vi "ADAM_scan_table.vi"() -> ()   [LabVIEW 2012]
uses:
  Anemometry/Anemometry Sub Vis/Controls/Serveds.ctl
  ADAM Client/Sub VIs/ADAM Controls/Module_type_ADAM.ctl
  ADAM Client/Sub VIs/ADAM Controls/Traverse_Level_State.ctl
  Anemometry/Anemometry Sub Vis/Controls/Post_Process.ctl
  ADAM Client/Sub VIs/ADAM Controls/Channel_State.ctl
  ADAM Client/Sub VIs/ADAM Controls/Ch_description_ADAM.ctl
  ADAM Client/Sub VIs/ADAM Controls/Function_ADAM.ctl
  ADAM Client/Sub VIs/ADAM Controls/Calib_type_ADAM.ctl
  ADAM Client/Sub VIs/ADAM Controls/Address.ctl
  ADAM_Global.vi
  Sub VI's/Channel_Description_Global.vi
  Anemometry/Anemometry Sub Vis/Globals/Meas_global.vi
  Sub VI's/Logged_Data_real_Global.vi
  Anemometry/Anemometry Sub Vis/Globals/Preference_global.vi
  Anemometry/Anemometry Sub Vis/Globals/Gas_management_global.vi
  Anemometry/Anemometry Sub Vis/Globals/Constants_global.vi
panel:
  in  "Reconfigure Gills":bool
  in  "Full Res Pathname":path
  in  "Log full Res Data":bool
  out "Duty No":u16 format="%.0b"
  in  "Save Current setup":bool=TRUE
  in  "Load setup from file":bool
  out "ADAM scan comments":string
  out "History length":i32=250
  in  "stop":bool
  out "Results":dbl[](array[numeric]) format="%.3f"
  out "Titles":string[](array[string])
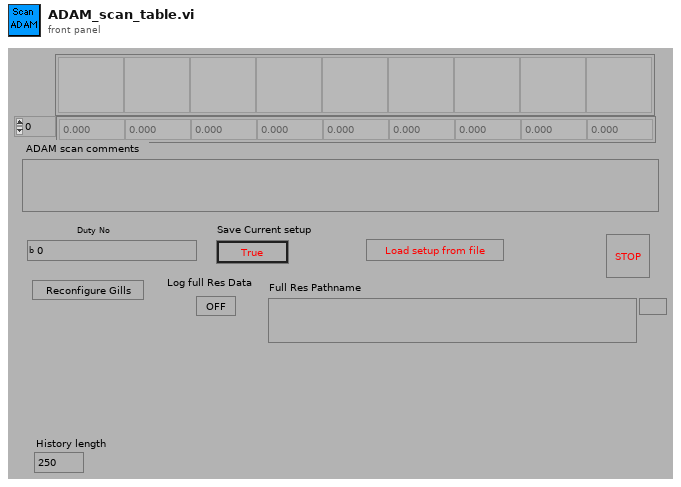
[diagram p1: front panel]
types:
  T1 = enum16{"Load ADAM setup from excel file", "Save ADAM setup to excel file"}
  T2 = typedef "Serveds.ctl" = enum16{"Read Global", "Load Global From File"}
  T3 = typedef "Module_type_ADAM.ctl" = string
  T4 = typedef "Traverse_Level_State.ctl" = enum16{"Running", "Complete"}
  T5 = typedef "Post_Process.ctl" = enum16{"Take New Data", "Post Process Raw Data File"}
  T6 = typedef "Channel_State.ctl" = enum16{"On", "Off", "Always On", "Always Off"}
  T7 = enum16{"Append to Global", "Read Global then Clear"}
  T8 = typedef "Ch_description_ADAM.ctl" = cluster{"Ch Name":string, "Type":T3, "Function":T9, "Ch State":T6, "Calibration type":T10, "A":dbl, "B":dbl, "C":dbl, "D":dbl, "Comments":string, "Address":T11, "String":string, "Duty":u16}
  T9 = typedef "Function_ADAM.ctl" = enum16{"Analogue Input", "Digital Input", "Event counter", "Event rate", "Analogue Output", "Digital Output", "Relay Output"}
  T10 = typedef "Calib_type_ADAM.ctl" = enum16{"Raw", "Bx + A", "Cx^2 + Bx + A", "Dx^3 + Cx^2 + Bx + A", "In Band", "Hi-Tec Q", "Hi-Tec M_dot", "Text"}
  T11 = typedef "Address.ctl" = cluster{"Main":i32, "Ch.":i32, "Sub":i32, "Port Name":string}
  T12 = typedef "Client_State_Cluster.ctl" = cluster{"Client Name":string, "Traverse level State":T4, "People to Email":string[], "Next Contact Time":dbl}
  T13 = typedef "ADAM_Comparitor.ctl" = cluster{"Ch to Monitor":string, "Channels to Kill":string, "Warn if Above":dbl, "Warn if Below":dbl, "Kill if Above":dbl, "Kill if Below":dbl, "Hysteresis Margin":dbl, "Averaging TIme (s)":dbl, "Warn Status":bool, "Kill Status":bool, "Extra Email addresses":string}
  T14 = typedef "Update_scan_value.ctl" = cluster{"Channel Name":string, "New Value":dbl}
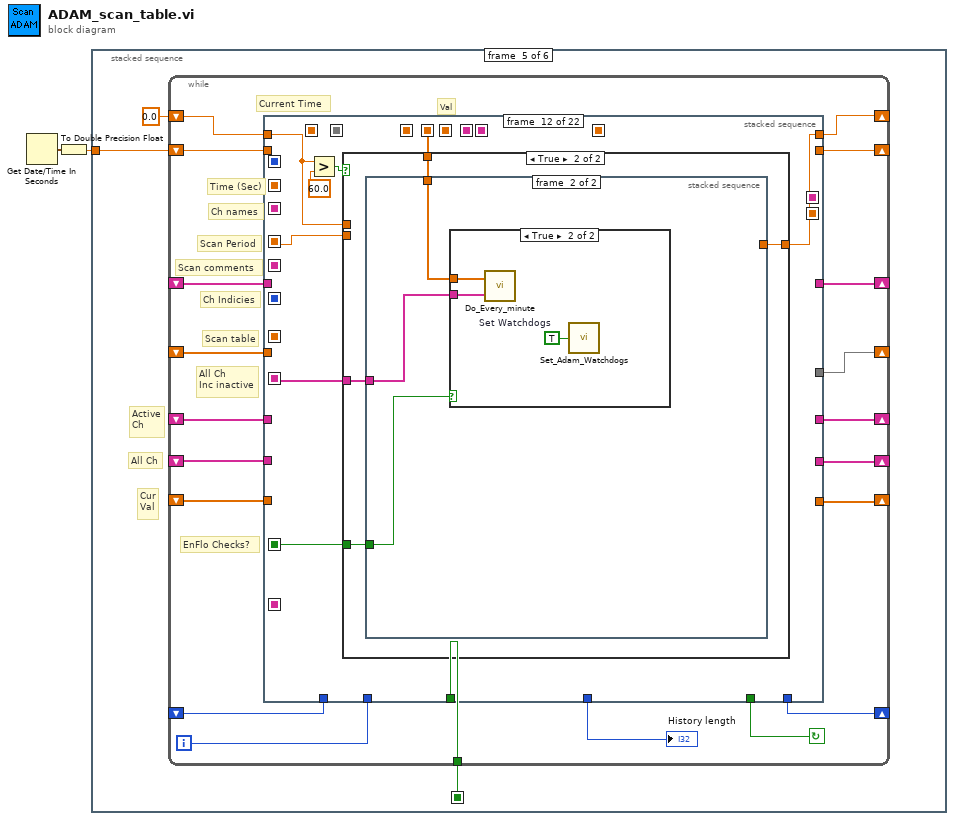
[diagram p0: block diagram]
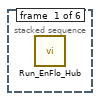
[diagram p2: hidden frame]
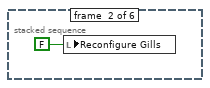
[diagram p3: hidden frame]
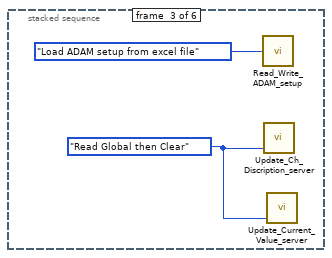
[diagram p4: hidden frame]
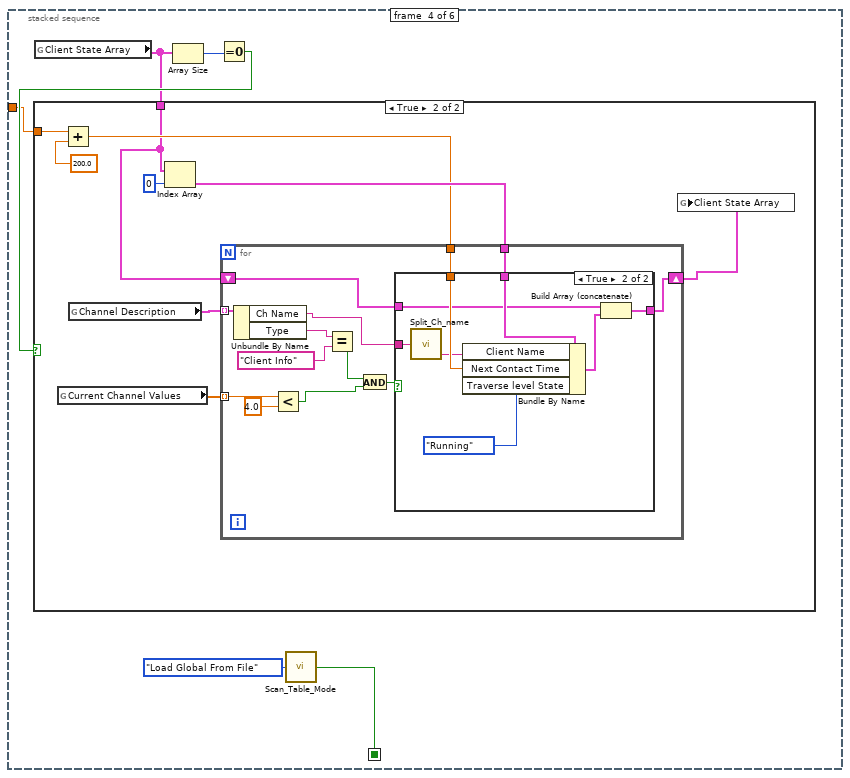
[diagram p5: hidden frame]
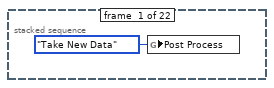
[diagram p8: hidden frame]
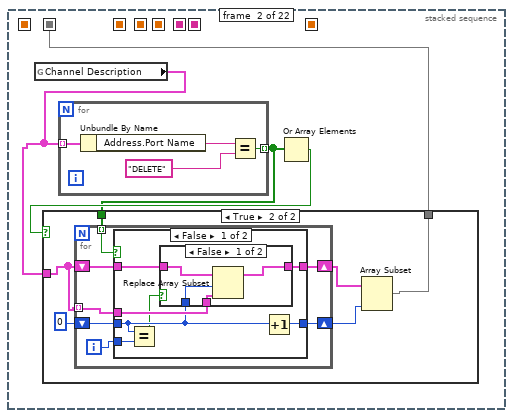
[diagram p9: hidden frame]
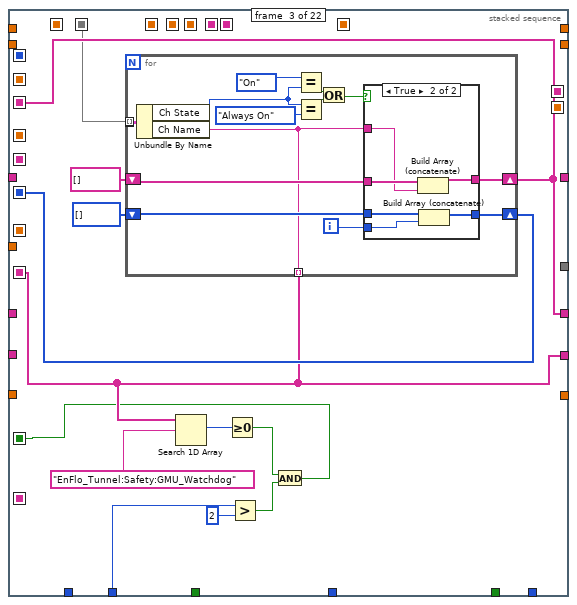
[diagram p13: hidden frame]
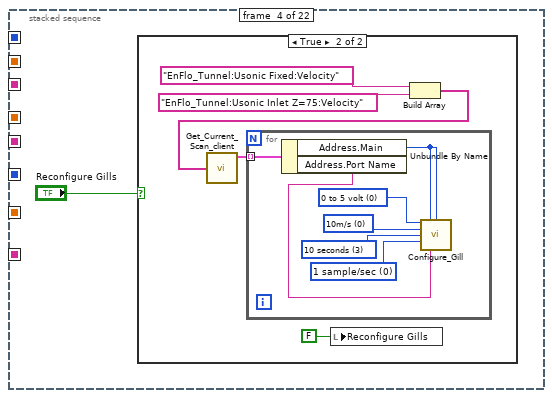
[diagram p15: hidden frame]
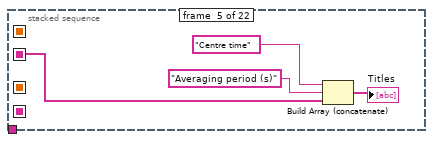
[diagram p17: hidden frame]
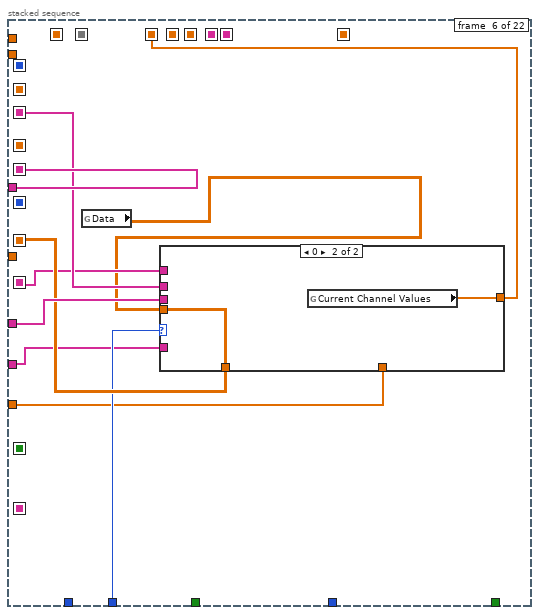
[diagram p18: hidden frame]
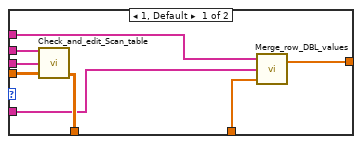
[diagram p19: hidden frame]
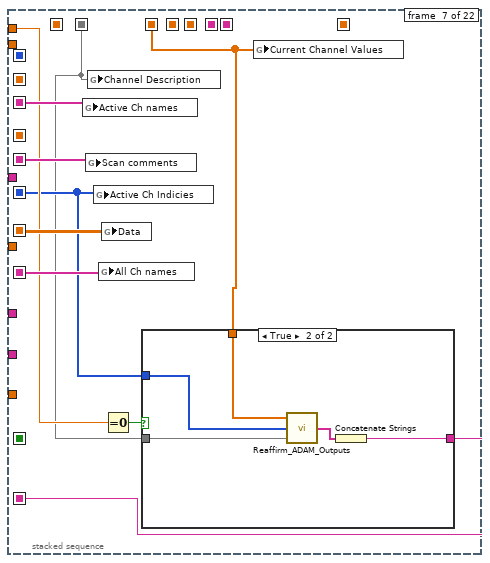
[diagram p20: hidden frame]
diagram:
  n1 = Get Date/Time In Seconds() -> (seconds since 1Jan1904=w2:timestamp)
  n2 = To Double Precision Float(number=w2) -> (double precision float=w1:dbl)
  n3 = stacked-sequence {
    seq-local: [_ _ _ w11 _ _] -> [_ _ _ _ w45 _]
    tunnel: w1 -> [_ _ _ w6 w43 _]
    frame #0 {
      n4 = call "Run_EnFlo_Hub.vi"() -> ()  [unwired: 8 out]
    }
    frame #1 {
      n5 = local write "Reconfigure Gills"(FALSE ("Reconfigure Gills")) -> ()
    }
    frame #2 {
      w4 = T7."Read Global then Clear" ("Mode")
      n6 = call "Read_Write_ADAM_setup.vi"("Mode"=T1."Load ADAM setup from excel file") -> ()  [unwired: 4 out]
      n7 = call "Update_Ch_Discription_server.vi"("Mode"=w4) -> ()  [unwired: 2 in, 1 out]
      n8 = call "Update_Current_Value_server.vi"("Mode"=w4) -> ()  [unwired: 2 in, 1 out]
    }
    frame #3 {
      n9 = global read "ADAM_Global.vi" "Client State Array"() -> (w7:T12[])
      n10 = Array Size(array=w7) -> (size(s)=w9:i32)
      n11 = Equal To 0?(x=w9) -> (x = 0?=w8:bool)
      n12 = case shown="True" w8 {
        tunnel: w7 -> [_ w13]
        tunnel: w6 -> [_ w16]
        frame False {
        }
        frame True {
          n13 = global read "ADAM_Global.vi" "Current Channel Values"() -> (w20:dbl[])
          n14 = Add(x=w16, y=200.0) -> (x+y=w14:dbl)
          n15 = global read "Channel_Description_Global.vi" "Channel Description"() -> (w19:T8[])
          n16 = Index Array(array=w13, index=0) -> (element=w17:T12)
          n17 = for {
            tunnel: w19 -> [w33] mode=indexing
            tunnel: w20 -> [w25] mode=indexing
            tunnel: w17 -> [w26]
            tunnel: w14 -> [w24]
            shift-right: [w23] -> w12
            shift-left: w13 -> [w22]
            n18 = Unbundle By Name(w33) -> ("Ch Name"=w21:string, "Type"=w30:T3)
            n19 = Less?(x=w25, y=4.0) -> (x < y?=w28:bool)
            n20 = Equal?(x=w30, y=T3 "Client Info" ("Type")) -> (x = y?=w29:bool)
            n21 = And(x=w29, y=w28) -> (x .and. y?=w27:bool)
            n22 = case shown="True" w27 {
              tunnel: w26 -> [_ w42]
              tunnel: w24 -> [_ w41]
              tunnel: [w34 w39] -> w23
              tunnel: w22 -> [w34 w38]
              tunnel: w21 -> [_ w36]
              frame False {
              }
              frame True {
                n23 = call "Split_Ch_name.vi"("Ch name"=w36) -> ("Low level"=w35:string)  [unwired: 2 out]
                n24 = Bundle By Name(cluster=w42, "Client Name"=w35, "Next Contact Time"=w41, "Traverse level State"=Traverse_Level_State."Running") -> (w37:T12)
                n25 = Build Array (concatenate)(w38, w37) -> (w39:T12[])
              }
            }
          }
          n26 = global write "ADAM_Global.vi" "Client State Array"(w12) -> ()
        }
      }
      n27 = call "Scan_Table_Mode.vi"("Mode"=Serveds."Load Global From File") -> ("Simulate Mode ?"=w11:bool)
    }
    frame #4 {
      # "Active\nCh"
      # "Cur\nVal"
      # "All Ch"
      n28 = while {
        shift-left: _ -> [w47]
        shift-right: [w46] -> _
        shift-left: _ -> [w48]
        shift-right: [w49] -> _
        shift-left: _ -> [w50]
        shift-right: [w51] -> _
        tunnel: w45 -> [w53]
        shift-left: _ -> [w56]
        shift-right: [w55] -> _
        shift-left: 0.0 -> [w57]
        shift-right: [w52] -> _
        shift-left: _ -> [w59]
        shift-right: [w60] -> _
        shift-left: _ -> [w61]
        shift-right: [w62] -> _
        shift-left: w43 -> [w63]
        shift-right: [w64] -> _
        i -> [w58]
        stop <- w65 continue-if-true
        # "Current Time"
        # "EnFlo Checks?"
        # "Val"
        # "All Ch\nInc inactive"
        # "Scan comments"
        # "Scan table"
        # "Time (Sec)"
        # "Ch Indicies"
        # "Ch names"
        # "Scan Period"
        n29 = stacked-sequence {
          seq-local: [_ _ _ _ _ _ _ _ _ _ _ _ w300 _ _ _ _ _ _ _ _ _] -> [_ _ _ _ _ _ _ _ _ _ _ _ _ _ w351 w356 _ _ _ _ w434 _]
          seq-local: [_ _ _ _ _ _ _ w193 _ _ _ _ _ _ _ _ _ _ _ _ _ _] -> [_ _ _ _ _ _ _ _ _ _ _ _ _ _ _ w363 _ _ _ _ _ _]
          seq-local: [_ _ _ _ _ w160 _ _ _ _ _ _ _ _ _ _ _ _ _ _ _ _] -> [_ _ _ _ _ _ w180 _ _ _ _ _ _ _ _ w361 _ _ _ _ _ _]
          seq-local: [_ _ _ _ _ _ _ w197 _ _ _ _ _ _ _ _ _ _ _ _ _ _] -> [_ _ _ _ _ _ _ _ _ w220 _ w266 _ _ _ w362 _ _ _ _ _ _]
          seq-local: [_ _ _ _ _ w163 _ _ _ _ _ _ _ _ _ _ _ _ _ _ _ _] -> [_ _ _ _ _ _ w182 _ _ _ _ _ _ _ _ _ _ w401 _ _ _ _]
          seq-local: [_ _ _ _ _ _ _ _ _ w218 _ _ _ _ _ _ _ _ _ _ _ _] -> [_ _ _ _ _ _ _ _ _ _ w237 _ _ _ _ _ _ _ _ _ _ _]
          seq-local: [_ _ w114 _ _ _ _ _ _ _ _ _ _ _ _ _ _ _ _ _ _ _] -> [_ _ _ _ w152 w162 w183 w198 _ _ _ _ _ _ _ w359 w364 _ _ _ _ _]
          seq-local: [_ _ w113 _ _ _ _ _ _ _ _ _ _ _ _ _ _ _ _ _ _ _] -> [_ _ _ _ _ _ w176 _ _ w219 _ _ _ _ _ _ _ _ _ _ _ _]
          seq-local: [_ _ _ _ _ w156 _ _ _ _ _ _ _ _ _ _ _ _ _ _ _ _] -> [_ _ _ _ _ _ w177 _ _ w216 _ _ _ _ _ _ _ _ _ _ _ _]
          seq-local: [_ _ _ _ _ _ _ _ _ w214 _ _ _ _ _ _ _ _ _ _ _ _] -> [_ _ _ _ _ _ _ _ _ _ w242 w265 w298 _ _ _ _ _ _ _ _ _]
          seq-local: [_ _ w109 _ _ _ _ _ _ _ _ _ _ _ _ _ _ _ _ _ _ _] -> [_ _ _ _ _ w158 w181 _ _ w215 w241 w264 w299 w324 w343 w358 _ _ _ w411 _ _]
          seq-local: [_ _ _ _ _ _ _ _ w200 _ _ _ _ _ _ _ _ _ _ _ _ _] -> [_ _ _ _ _ _ _ _ _ w213 _ _ _ _ _ _ _ _ _ _ _ _]
          seq-local: [_ w67 _ _ _ _ _ _ _ _ _ _ _ _ _ _ _ _ _ _ _ _] -> [_ _ w111 _ _ _ w175 _ _ w212 _ _ _ _ _ _ _ _ _ _ _ _]
          seq-local: [_ _ _ _ _ _ _ w192 _ _ _ _ _ _ _ _ _ _ _ _ _ _] -> [_ _ _ _ _ _ _ _ _ _ w238 _ _ _ _ _ w366 _ _ _ _ _]
          seq-local: [_ _ _ _ _ _ _ _ _ _ _ _ _ _ _ w355 _ _ _ _ _ _] -> [_ _ _ _ _ _ _ _ _ _ _ _ _ _ _ _ w365 _ _ _ _ _]
          seq-local: [_ _ w103 _ _ _ _ _ _ _ _ _ _ _ _ _ _ _ _ _ _ _] -> [_ _ _ _ _ _ _ w190 _ _ w240 w263 _ _ _ _ _ _ _ _ _ w438]
          seq-local: [_ _ _ _ _ _ _ _ _ _ _ _ w297 _ _ _ _ _ _ _ _ _] -> [_ _ _ _ _ _ _ _ _ _ _ _ _ w325 _ _ _ _ _ _ _ _]
          seq-local: [_ _ _ _ _ _ w174 _ _ _ _ _ _ _ _ _ _ _ _ _ _ _] -> [_ _ _ _ _ _ _ _ _ w211 _ _ _ _ _ _ _ _ _ _ _ _]
          seq-local: [_ _ _ _ _ _ _ _ _ _ _ _ w296 _ _ _ _ _ _ _ _ _] -> [_ _ _ _ _ _ _ _ _ _ _ _ _ w323 _ _ _ _ _ _ _ _]
          seq-local: [_ _ _ _ _ _ _ _ _ _ w236 _ _ _ _ _ _ _ _ _ _ _] -> [_ _ _ _ _ _ _ _ _ _ _ _ _ _ _ _ _ w389 _ _ _ _]
          tunnel: [_ _ _ _ _ _ _ _ _ _ _ _ _ _ _ _ _ _ w409 _ _ _] -> w65
          tunnel: [_ _ _ _ _ _ _ w192 _ _ _ _ _ _ _ _ _ _ _ _ _ _] -> w64
          tunnel: w63 -> [_ _ _ _ _ _ _ w194 _ _ _ _ _ _ _ _ _ _ _ _ _ _]
          tunnel: [_ _ _ _ _ _ _ _ _ _ _ _ _ _ _ _ _ w399 _ _ _ _] -> w62
          tunnel: w61 -> [_ _ _ _ _ w163 _ _ _ _ _ _ _ _ _ _ _ _ _ _ _ _]
          tunnel: [_ _ w114 _ _ _ _ _ _ _ _ _ _ _ _ _ _ _ _ _ _ _] -> w60
          tunnel: w59 -> [_ _ _ _ _ w161 _ _ _ _ _ _ _ w326 _ _ _ _ _ _ _ _]
          tunnel: w58 -> [_ _ w107 _ _ w159 _ _ _ _ w239 _ _ _ _ _ _ _ w407 _ _ w439]
          tunnel: w57 -> [_ _ _ _ _ _ w178 _ _ _ _ w268 _ _ _ _ _ _ _ _ _ _]
          tunnel: [_ _ _ _ _ _ _ _ _ _ _ w270 _ _ _ _ _ _ _ _ _ _] -> w52
          tunnel: w56 -> [_ _ _ _ _ _ _ _ _ _ _ _ _ _ w349 _ _ _ _ _ _ _]
          tunnel: [_ _ _ _ _ _ _ _ _ _ _ _ _ _ w345 _ _ _ _ _ _ _] -> w55
          tunnel: [_ _ _ _ _ _ _ _ _ _ _ _ _ _ _ w360 _ _ _ _ _ _] -> w54
          tunnel: w53 -> [_ _ _ _ _ _ _ _ _ w217 _ _ _ _ _ _ _ _ _ _ _ _]
          tunnel: [_ _ w109 _ _ _ _ _ _ _ _ _ _ _ _ _ _ _ _ _ _ _] -> w51
          tunnel: w50 -> [_ _ _ _ _ w157 _ _ _ _ _ _ _ _ _ _ _ _ _ _ _ _]
          tunnel: [_ _ _ _ _ _ _ _ _ _ _ _ _ _ _ _ _ _ _ _ w434 _] -> w49
          tunnel: w48 -> [_ _ _ _ _ w155 _ _ _ _ _ _ _ _ _ _ _ _ _ _ _ _]
          tunnel: w47 -> [_ _ _ _ _ _ _ _ w201 _ _ _ _ _ _ _ _ _ _ _ _ _]
          tunnel: [_ _ _ _ _ _ _ _ w202 _ _ _ _ _ _ _ _ _ _ _ _ _] -> w46
          frame #0 {
            n30 = global write "Meas_global.vi" "Post Process"(Post_Process."Take New Data" ("Post Process")) -> ()
          }
          frame #1 {
            n31 = global read "Channel_Description_Global.vi" "Channel Description"() -> (w69:T8[])
            n32 = for {
              tunnel: w69 -> [w102] mode=indexing
              tunnel: [w99] -> w68 mode=indexing
              n33 = Unbundle By Name(w102) -> ("Address.Port Name"=w101:string)
              n34 = Equal?(x=w101, y="DELETE") -> (x = y?=w99:bool)
            }
            n35 = Or Array Elements(Boolean array=w68) -> (logical OR=w70:bool)
            n36 = case shown="True" w70 {
              tunnel: w69 -> [w71 w75]
              tunnel: w68 -> [_ w77]
              tunnel: [w71 w72] -> w67
              frame False {
              }
              frame True {
                n37 = for {
                  shift-right: [w84] -> w74
                  shift-left: w75 -> [w83]
                  tunnel: w77 -> [w79] mode=indexing
                  shift-right: [w82] -> w73
                  shift-left: 0 -> [w80]
                  tunnel: w75 -> [w81] mode=indexing
                  i -> [w78]
                  n38 = case shown="False" w79 {
                    tunnel: [w90 w98] -> w84
                    tunnel: w83 -> [w91 w98]
                    tunnel: [w88 w97] -> w82
                    tunnel: w80 -> [w87 w97]
                    tunnel: w81 -> [w89 _]
                    tunnel: w78 -> [w86 _]
                    frame False {
                      n39 = Equal?(x=w87, y=w86) -> (x = y?=w85:bool)
                      n40 = case shown="False" w85 {
                        tunnel: w91 -> [w95 w96]
                        tunnel: [w94 w96] -> w90
                        tunnel: w89 -> [w93 _]
                        tunnel: w87 -> [w92 _]
                        frame False {
                          n41 = Replace Array Subset(array=w95, new element=w93, index=w92) -> (w94:T8[])
                        }
                        frame True {
                        }
                      }
                      n42 = Increment(x=w87) -> (x+1=w88:i32)
                    }
                    frame True {
                    }
                  }
                }
                n43 = Array Subset(array=w74, length=w73) -> (w72:T8[])  [unwired: 1 in]
              }
            }
          }
          frame #2 {
            n44 = for {
              tunnel: [w128] -> _ mode=indexing
              shift-right: [w127] -> w114
              shift-left: string[] [] -> [w118]
              shift-right: [w124] -> w113
              shift-left: i32[] [] -> [w126]
              tunnel: [w116] -> w109 mode=indexing
              tunnel: w111 -> [w128] mode=indexing
              i -> [w125]
              n45 = Unbundle By Name(w128) -> ("Ch State"=w119:T6, "Ch Name"=w116:string)
              n46 = Equal?(x=Channel_State."On" ("Channel State"), y=w119) -> (x = y?=w121:bool)
              n47 = Equal?(x=w119, y=Channel_State."Always On" ("Channel State")) -> (x = y?=w120:bool)
              n48 = Or(x=w121, y=w120) -> (x .or. y?=w117:bool)
              n49 = case shown="True" w117 {
                tunnel: w118 -> [w129 w136]
                tunnel: w116 -> [_ w135]
                tunnel: [w129 w134] -> w127
                tunnel: w126 -> [w130 w133]
                tunnel: w125 -> [_ w132]
                tunnel: [w130 w131] -> w124
                frame False {
                }
                frame True {
                  n50 = Build Array (concatenate)(w136, w135) -> (w134:string[])
                  n51 = Build Array (concatenate)(w133, w132) -> (w131:i32[])
                }
              }
            }
            n52 = Search 1D Array(1D array=w109, element="EnFlo_Tunnel:Safety:GMU_Watchdog") -> (index of element=w108:i32)  [unwired: 1 out]
            n53 = Greater Or Equal To 0?(x=w108) -> (x >= 0?=w104:bool)
            n54 = Greater?(x=w107, y=2) -> (0:w105:bool)
            n55 = And(x=w104, y=w105) -> (x .and. y?=w103:bool)
          }
          frame #3 {
            n56 = case shown="True" "Reconfigure Gills" {
              frame False {
              }
              frame True {
                n57 = local write "Reconfigure Gills"(FALSE ("Reconfigure Gills")) -> ()
                n58 = Build Array("EnFlo_Tunnel:Usonic Fixed:Velocity", "EnFlo_Tunnel:Usonic Inlet Z=75:Velocity") -> (w140:string[])
                n59 = call "Get_Current_Scan_client.vi"("ADAM Ch Names"=w140) -> ("Ch Description Array"=w139:T8[])  [unwired: 3 out]
                n60 = for {
                  tunnel: w139 -> [w145] mode=indexing
                  w149 = u16 0 items=["1 sample/sec", "4 samples/sec"] ("Samples/sec")
                  w148 = u16 3 items=["OFF", "3 seconds", "5 seconds", "10 seconds"] ("Averaging Time")
                  w147 = u16 0 items=["10m/s", "20m/s", "30m/s", "40m/s", "50m/s", "60m/s", "70m/s"] ("Analogue O/P Scale")
                  w146 = u16 0 items=["0 to 5 volt", "+/-2.5 Volt", "4-20mA"] ("Analogue O/P Config")
                  n61 = Unbundle By Name(w145) -> ("Address.Main"=w144:i32, "Address.Port Name"=w143:string)
                  n62 = call "Configure_Gill.vi"("Analogue O/P Config"=w146, "ORIGINAL Address"=w144, "NEW Address"=w144, "Analogue O/P Scale"=w147, "Averaging Time"=w148, "Samples/sec"=w149, "Port Name"=w143) -> ()  [unwired: 9 out]
                }
              }
            }
          }
          frame #4 {
            n63 = Build Array (concatenate)("Centre time", "Averaging period (s)", w152) -> (→"Titles":string[])
          }
          frame #5 {
            n64 = global read "Logged_Data_real_Global.vi" "Data"() -> (w154:dbl[][])
            n65 = case shown="0" w159 {
              tunnel: w154 -> [w171 w173]
              tunnel: w162 -> [w168 _]
              tunnel: w161 -> [w170 _]
              tunnel: [w169 w173] -> w160
              tunnel: w158 -> [w167 _]
              tunnel: w157 -> [w166 _]
              tunnel: [w165 w172] -> w156
              tunnel: w155 -> [w164 _]
              frame 1, Default {
                n66 = call "Check_and_edit_Scan_table.vi"("2D array input"=w171, "Original Channels"=w170, "Present Channels"=w168) -> ("2D array output"=w169:dbl[][])  [unwired: 2 out]
                n67 = call "Merge_row_DBL_values.vi"("Present Row values"=w164, "Present Channels"=w166, "Desired Channels"=w167) -> ("Desired Row values"=w165:dbl[])  [unwired: 1 out]
              }
              frame 0 {
                n68 = global read "ADAM_Global.vi" "Current Channel Values"() -> (w172:dbl[])
              }
            }
          }
          frame #6 {
            n69 = global write "ADAM_Global.vi" "Active Ch names"(w183) -> ()
            n70 = global write "ADAM_Global.vi" "Scan comments"(w182) -> ()
            n71 = global write "Channel_Description_Global.vi" "Channel Description"(w175) -> ()
            n72 = global write "ADAM_Global.vi" "Active Ch Indicies"(w176) -> ()
            n73 = global write "ADAM_Global.vi" "All Ch names"(w181) -> ()
            n74 = global write "Logged_Data_real_Global.vi" "Data"(w180) -> ()
            n75 = Equal To 0?(x=w178) -> (x = 0?=w179:bool)
            n76 = case shown="True" w179 {
              tunnel: w177 -> [_ w189]
              tunnel: w176 -> [_ w188]
              tunnel: w175 -> [_ w187]
              tunnel: ["" w185] -> w174
              frame False {
              }
              frame True {
                n77 = call "Reaffirm_ADAM_Outputs.vi"("Channel Description"=w187, "Active Ch Indicies"=w188, "Current Channel Values"=w189) -> ("Scan Comments"=w186:string[])  [unwired: 2 out]
                n78 = Concatenate Strings(w186) -> (w185:string)
              }
            }
            n79 = global write "ADAM_Global.vi" "Current Channel Values"(w177) -> ()
          }
          frame #7 {
            n80 = case shown="True" w190 {
              tunnel: w198 -> [_ w199]
              frame False {
              }
              frame True {
                n81 = call "Gas_Status_panel.vi"("Ch names"=w199) -> ()  [unwired: 15 out]
              }
            }
            n82 = Get Date/Time In Seconds() -> (seconds since 1Jan1904=w191:timestamp)
            n83 = To Double Precision Float(number=w191) -> (double precision float=w192:dbl)
            n84 = Subtract(x=w192, y=w194) -> (x-y=w197:dbl)
            n85 = Divide(x=w197, y=2.0) -> (x/y=w195:dbl)
            n86 = Add(x=w195, y=w194) -> (x+y=w193:dbl)
          }
          frame #8 {
            n87 = Equal To 0?(x=w201) -> (x = 0?=w205:bool)
            n88 = Equal?(x=u16 32768, y=w201) -> (x = y?=w204:bool)
            n89 = Select(t=u16 1, s=w205, f=w201) -> (s? t:f=w200:u16)
            "Duty No" <- w200
            n90 = case shown="False" w204 {
              tunnel: [w207 u16 0] -> w202
              tunnel: w200 -> [w209 _]
              frame False {
                n91 = Multiply(x=u16 2, y=w209) -> (x*y=w207:u16)
              }
              frame True {
              }
            }
          }
          frame #9 {
            n92 = for {
              tunnel: w212 -> [w227]
              tunnel: w220 -> [w235]
              shift-right: [w233] -> w214
              shift-left: w216 -> [w231]
              tunnel: w215 -> [w232]
              shift-right: [w228] -> w218
              shift-left: w211 -> [w230]
              tunnel: w219 -> [w222] mode=indexing
              tunnel: w216 -> [w224]
              tunnel: w217 -> [w225]
              tunnel: w213 -> [w221]
              n93 = Index Array(array=w224, index=w222) -> (element=w223:dbl)
              n94 = Index Array(array=w227, index=w222) -> (element=w226:T8)
              n95 = call "Adam_Ch_Input_Output.vi"("Simulate"=w225, "Duty No"=w221, "Previuos Scan Value"=w223, "Ch values"=w231, "Scan Period"=w235, "Ch Discription"=w226, "Ch names"=w232) -> ("Scan comment"=w229:string, "Calibrated units"=w234:dbl)  [unwired: 1 in, 2 out]
              n96 = Concatenate Strings(w230, w229) -> (w228:string)
              n97 = Replace Array Subset(array=w231, new element=w234, index=w222) -> (w233:dbl[])
            }
          }
          frame #10 {
            n98 = case shown="True" w240 {
              tunnel: w242 -> [_ w249]
              tunnel: w241 -> [_ w248]
              tunnel: w239 -> [_ w247]
              tunnel: w238 -> [_ w257]
              tunnel: w237 -> [w244 w246]
              tunnel: [w244 w254] -> w236
              frame False {
              }
              frame True {
                n99 = global read "ADAM_Global.vi" "Comparitor Array"() -> (w253:T13[])
                n100 = for {
                  tunnel: w253 -> [w262] mode=indexing
                  tunnel: [w261] -> w252 mode=indexing
                  tunnel: w249 -> [w260]
                  tunnel: w248 -> [w259]
                  tunnel: [w258] -> w251 mode=indexing
                  n101 = call "ADAM_Comparitor.vi"("Comparator Info"=w262, "Ch names"=w259, "Present scan array"=w260) -> ("Comparator Info Out"=w261:T13, "Scan comment"=w258:string)  [unwired: 1 in]
                }
                n102 = call "LDA1_Safety.vi"("Adam Loop Count"=w247, "Ch Names"=w248, "Values"=w249) -> ("Scan comment"=w245:string)
                n103 = call "LDA2_Safety.vi"("Adam Loop Count"=w247, "Ch Names"=w248, "Values"=w249) -> ("Scan comment"=w250:string)
                n104 = call "Safety_Check.vi"("Adam Loop Count"=w247, "Ch Names"=w248, "Values"=w249) -> ("Scan comment"=w256:string)
                n105 = call "Check_Aero_Tunnel_on_Server.vi"("Values"=w249, "Ch Names"=w248, "Current Time"=w257, "Adam Loop Count"=w247) -> ("Scan comment"=w255:string)  [unwired: 2 in]
                n106 = global write "ADAM_Global.vi" "Comparitor Array"(w252) -> ()
                n107 = Concatenate Strings(w246, w245, w250, w256, w255, w251) -> (w254:string)
              }
            }
            n108 = property on="Results" class="Arr (strict)"() -> ("Index Values"=w243:u32[])  [unwired: 2 in, 2 out]
            n109 = property on="Titles" class="Arr (strict)"("Index Values"=w243) -> ()  [unwired: 2 in, 2 out]
          }
          frame #11 {
            n110 = Greater?(x=w268, y=60.0) -> (0:w269:bool)
            n111 = case shown="True" w269 {
              tunnel: [w272 w277] -> w270
              tunnel: w268 -> [w273 _]
              tunnel: w266 -> [w271 _]
              tunnel: w265 -> [_ w276]
              tunnel: w264 -> [_ w275]
              tunnel: w263 -> [_ w274]
              frame False {
                n112 = Add(x=w273, y=w271) -> (x+y=w272:dbl)
              }
              frame True {
                n113 = stacked-sequence {
                  tunnel: [0.0 _] -> w277
                  tunnel: w276 -> [_ w292]
                  tunnel: w275 -> [_ w291]
                  tunnel: w274 -> [_ w290]
                  frame #0 {
                    n114 = case shown="False" "Save Current setup" {
                      tunnel: [FALSE w282] -> w278
                      frame False {
                      }
                      frame True {
                        n115 = Get Date/Time In Seconds() -> (seconds since 1Jan1904=w284:timestamp)
                        n116 = global read "ADAM_Global.vi" "Network Last checked"() -> (w288:dbl)
                        n117 = To Double Precision Float(number=w284) -> (double precision float=w283:dbl)
                        n118 = Subtract(x=w288, y=w283) -> (x-y=w287:dbl)
                        n119 = Absolute Value(x=w287) -> (abs(x)=w286:dbl)
                        n120 = Less?(x=w286, y=1.5) -> (x < y?=w282:bool)
                      }
                    }
                    n121 = case shown="True" w278 {
                      frame False {
                      }
                      frame True {
                        n122 = call "Read_Write_ADAM_setup.vi"("Mode"=T1."Save ADAM setup to excel file") -> ()  [unwired: 4 out]
                      }
                    }
                  }
                  frame #1 {
                    n123 = case shown="True" w290 {
                      tunnel: w292 -> [_ w295]
                      tunnel: w291 -> [_ w294]
                      frame False {
                      }
                      frame True {
                        w293 = TRUE  # Set Watchdogs
                        n124 = call "Do_Every_minute.vi"("Ch Names"=w294, "Values"=w295) -> ()  [unwired: 1 out]
                        n125 = call "Set_Adam_Watchdogs.vi"("Set Watchdogs"=w293) -> ()  [unwired: 1 out]
                      }
                    }
                  }
                }
              }
            }
          }
          frame #12 {
            n126 = call "Update_Current_Value_server.vi"("Mode"=T7."Read Global then Clear") -> ("Update array out"=w302:T14[])  [unwired: 2 in]
            n127 = for {
              tunnel: w299 -> [w310]
              tunnel: w302 -> [w305] mode=indexing
              shift-right: [w308] -> w300
              shift-left: w298 -> [w309]
              tunnel: [w304] -> w297 mode=indexing
              tunnel: [w303] -> w296 mode=indexing
              n128 = Unbundle By Name(w305) -> ("Channel Name"=w304:string, "New Value"=w303:dbl)
              n129 = Search 1D Array(1D array=w310, element=w304) -> (index of element=w307:i32)  [unwired: 1 out]
              n130 = Less Than 0?(x=w307) -> (x < 0?=w306:bool)
              n131 = case shown="True" w306 {
                tunnel: w304 -> [_ w311]
                tunnel: w305 -> [_ w316]
                frame False {
                }
                frame True {
                  n132 = global read "ADAM_Global.vi" "Update Current Value"() -> (w315:T14[])
                  n133 = call "Check_Ch_Name_colons.vi"("No of Colons"=2, "Ch Name in"=w311) -> ("Ch Name out"=w312:string)
                  n134 = Bundle By Name(cluster=T8 {"Ch Name"="", "Type"="Hold Value", "Function"=enum."Analogue Input", "Ch State"=enum."On", "Calibration type"=enum."Raw", "A"=0.0, "B"=0.0, "C"=0.0, "D"=0.0, "Comments"="", "Address"={"Main"=0, "Ch."=0, "Sub"=0, "Port Name"=""}, "String"="", "Duty"=0} ("Ch Description"), "Ch Name"=w312, "Type"=T3 "Hold Value") -> (w320:T8)
                  n135 = Build Array (concatenate)(w315, w316) -> (w314:T14[])
                  n136 = global write "ADAM_Global.vi" "Update Current Value"(w314) -> ()
                  n137 = global read "Preference_global.vi" "Rig Setup"() -> (w318:string)
                  n138 = Build Array(w320) -> (w319:T8[])
                  n139 = call "Update_Ch_Discription_server.vi"("Mode"=T7."Append to Global", "Client HD name"=w318, "Channels to update In"=w319) -> ()  [unwired: 1 out]
                }
              }
              n140 = Replace Array Subset(array=w309, new element=w303, index=w307) -> (w308:dbl[])
            }
          }
          frame #13 {
            n141 = for {
              tunnel: w326 -> [w334]
              tunnel: w325 -> [w332] mode=indexing
              tunnel: w324 -> [w333]
              tunnel: w323 -> [w330] mode=indexing
              n142 = Search 1D Array(1D array=w334, element=w332) -> (index of element=w331:i32)  [unwired: 1 out]
              n143 = Less Than 0?(x=w331) -> (x < 0?=w329:bool)
              n144 = Not Equal To 0?(x=w330) -> (x != 0?=w328:bool)
              n145 = And(x=w328, y=w329) -> (x .and. y?=w327:bool)
              n146 = case shown="True" w327 {
                tunnel: w333 -> [_ w342]
                tunnel: w332 -> [_ w341]
                frame False {
                }
                frame True {
                  n147 = Search 1D Array(1D array=w342, element=w341) -> (index of element=w336:i32)  [unwired: 1 out]
                  n148 = global read "Channel_Description_Global.vi" "Channel Description"() -> (w337:T8[])
                  n149 = Index Array(array=w337, index=w336) -> (element=w340:T8)
                  n150 = Bundle By Name(cluster=w340, "Ch State"=Channel_State."On") -> (w338:T8)
                  n151 = Replace Array Subset(array=w337, new element=w338, index=w336) -> (w335:T8[])
                  n152 = global write "Channel_Description_Global.vi" "Channel Description"(w335) -> ()
                }
              }
            }
          }
          frame #14 {
            n153 = Search 1D Array(1D array=w343, element="GMU:Source:Release Temp") -> (index of element=w350:i32)  [unwired: 1 out]
            n154 = Index Array(array=w351, index=w350) -> (element=w348:dbl)
            n155 = Build Array (concatenate)(w348, w349) -> (w347:dbl[])
            n156 = Array Subset(array=w347, length=10 ("Array Length")) -> (w345:dbl[])  [unwired: 1 in]
            n157 = call "Mean_fr_NaN_data.vi"("Data"=w345) -> ("Mean value"=w344:dbl)  [unwired: 1 out]
            n158 = global write "Gas_management_global.vi" "Release temp (deg C)"(w344) -> ()
          }
          frame #15 {
            w353 = 250000  # Table size
            n159 = call "Merge_row_DBL_values.vi"("Present Row values"=w356, "Present Channels"=w358, "Desired Channels"=w359) -> ("Desired Row values"=w357:dbl[])  [unwired: 1 out]
            n160 = Build Array (concatenate)(w363, w362, w357) -> (w355:dbl[])
            "Results" <- w355
            n161 = call "Manipulate_Table.vi"("Table size"=w353, "Latest Row"=w355, "Table Input"=w361) -> ("History length"=w360:i32, "Table Output"=w354:dbl[][])  [unwired: 1 out]
            n162 = global write "Logged_Data_real_Global.vi" "Data"(w354) -> ()
          }
          frame #16 {
            n163 = case shown="True" "Log full Res Data" {
              tunnel: w366 -> [_ w379]
              tunnel: w365 -> [_ w378]
              tunnel: w364 -> [_ w377]
              frame False {
              }
              frame True {
                n164 = Build Array (concatenate)(w379, w378) -> (w376:dbl[])
                n165 = Number To Fractional String(number=w376) -> (F-format string=w374:string[])  [unwired: 3 out]
                n166 = call "Does_file_exist_(simple).vi"("Pathname"="Full Res Pathname") -> ("exists?"=w373:bool)
                n167 = Build Array (concatenate)("Current time", "Centre Time", "Averaging period (s)", w377) -> (w375:string[])
                n168 = case shown="False" w373 {
                  tunnel: w375 -> [w385 _]
                  tunnel: w374 -> [w384 w386]
                  tunnel: [w381 w387] -> w369
                  frame False {
                    n169 = Build Array(w385, w384) -> (w382:string[][])
                    n170 = Array To Spreadsheet String(array=w382, 3:"%s" ("format string")) -> (spreadsheet string=w381:string)  [unwired: 1 out]
                  }
                  frame True {
                    n171 = Array To Spreadsheet String(array=w386, 3:"%s" ("format string")) -> (spreadsheet string=w387:string)  [unwired: 1 out]
                  }
                }
                n172 = call "Write_File_Simple.vi"("append to file? (new file:F)"=TRUE, "character string"=w369, "file path"="Full Res Pathname") -> ()  [unwired: 2 out]
              }
            }
          }
          frame #17 {
            w397 = 150 ("length")
            w398 = 50  # History length
            n173 = String Subset(string=w389, length (rest)=w397) -> (substring=w391:string)  [unwired: 1 out]
            n174 = String Length(string=w391) -> (length=w396:i32)
            n175 = Equal?(x=w397, y=w396) -> (x = y?=w395:bool)
            n176 = Select(t=" Clipped ", s=w395, f="") -> (s? t:f=w392:string)
            n177 = Concatenate Strings(w392, w391) -> (w390:string)
            n178 = Build Array (concatenate)(w401, w390) -> (w400:string[])
            n179 = Array Size(array=w400) -> (size(s)=w403:i32)
            n180 = Subtract(x=w403, y=w398) -> (x-y=w402:i32)
            n181 = Array Subset(array=w400, index=w402) -> (w399:string[])  [unwired: 1 in]
            "ADAM scan comments" <- w389
          }
          frame #18 {
            n182 = Format Into String(format string="%s %d %s" ("Format String"), "\nScan No " ("Header message"), w407, "\r\n") -> (resulting string=w406:string)  [unwired: 2 in, 1 out]
            n183 = call "Write_out_serial_log.vi"("Header message"=w406) -> ()
            n184 = Not(x="stop") -> (.not. x?=w409:bool)
          }
          frame #19 {
            n185 = call "Update_Ch_Discription_server.vi"("Mode"=T7."Read Global then Clear") -> ("Channels to update Out"=w412:T8[])  [unwired: 2 in]
            n186 = Array Size(array=w412) -> (size(s)=w414:i32)
            n187 = Equal To 0?(x=w414) -> (x = 0?=w413:bool)
            n188 = case shown="False" w413 {
              tunnel: w411 -> [w419 _]
              tunnel: w412 -> [w418 _]
              frame False {
                n189 = global read "Channel_Description_Global.vi" "Channel Description"() -> (w417:T8[])
                n190 = for {
                  tunnel: w419 -> [w426]
                  tunnel: w418 -> [w423] mode=indexing
                  shift-right: [w422] -> w416
                  shift-left: w417 -> [w425]
                  n191 = Unbundle By Name(w423) -> ("Ch Name"=w424:string)
                  n192 = Search 1D Array(1D array=w426, element=w424) -> (index of element=w420:i32)  [unwired: 1 out]
                  n193 = Less Than 0?(x=w420) -> (x < 0?=w421:bool)
                  n194 = case shown="False" w421 {
                    tunnel: w425 -> [w430 w433]
                    tunnel: w423 -> [w429 w431]
                    tunnel: [w428 w432] -> w422
                    tunnel: w420 -> [w427 _]
                    frame False {
                      n195 = Replace Array Subset(array=w430, new element=w429, index=w427) -> (w428:T8[])
                    }
                    frame True {
                      n196 = Build Array (concatenate)(w433, w431) -> (w432:T8[])
                    }
                  }
                }
                n197 = global write "Channel_Description_Global.vi" "Channel Description"(w416) -> ()
              }
              frame True {
              }
            }
          }
          frame #20 {
            n198 = case shown="True" "Load setup from file" {
              frame False {
              }
              frame True {
                n199 = local write "Save Current setup"(TRUE ("Save Current setup")) -> ()
                n200 = call "Read_Write_ADAM_setup.vi"("Mode"=T1."Load ADAM setup from excel file") -> ()  [unwired: 4 out]
              }
            }
          }
          frame #21 {
            n201 = case shown="0" w439 {
              tunnel: w438 -> [_ _]
              frame 0 {
                n202 = global read "Constants_global.vi" "EnFlo SW Folder"() -> (w444:path)
                n203 = Build Path(base path=w444, name or relative path=path "ADAM Client/ADAM client VIs/Plot_Server_Data.vi") -> (appended path=w441:path)
                n204 = call "Load_Comparitor_Cluster.vi"() -> ()  [unwired: 12 in]
                n205 = Build Path(base path=w444, name or relative path=path "ADAM Server/Log_ADAM_scan_table.vi") -> (appended path=w442:path)
                n206 = Build Array(w442, w441) -> (w440:path[])
                n207 = for {
                  tunnel: w440 -> [w446] mode=indexing
                  n208 = Open VI Reference(vi path=w446) -> (vi reference=w450:refnum<vi>, error out=w449:errorcluster)  [unwired: 2 in, 3 out]
                  n209 = property class="VI"(reference=w450, error in=w449, "Front Panel Window:Open"=TRUE) -> (reference out=w447:refnum<vi>, error out=w448:errorcluster)
                  n210 = invoke class="VI" method="Run VI"(reference=w447, error in=w448, "Wait until done"=FALSE) -> (reference out=w454:refnum<vi>, error out=w453:errorcluster)  [unwired: 2 in, 3 out]
                  n211 = Close Reference(reference=w454, error in (no error)=w453) -> ()  [unwired: 1 out]
                }
              }
              frame 1, Default {
              }
            }
          }
        }
        "History length" <- w54
      }
    }
    frame #5 {
      w455 = FALSE  # Set Watchdogs
      n212 = call "Set_Adam_Watchdogs.vi"("Set Watchdogs"=w455) -> ()  [unwired: 1 out]
      n213 = call "Read_Write_ADAM_setup.vi"("Mode"=T1."Save ADAM setup to excel file") -> ()  [unwired: 4 out]
    }
  }
